vi "Counter output test.vi"() -> ()   [LabVIEW 2013]
uses:
  <vilib>/DAQmx/create/channels.llb/DAQmx Create Channel (CO-Pulse Generation-Time).vi
  <vilib>/DAQmx/configure/timing.llb/DAQmx Timing (Implicit).vi
  <resource>/objmgr/daqmx.rc
panel:
  out "CO.Count":u32
  in  "counter":tag caption="计数器"
  in  "low time":dbl=0.01 caption="低时间" format="%.6f"
  in  "high time":dbl=0.01 caption="高时间" format="%.6f"
  in  "CO.Pulse.Term":tag
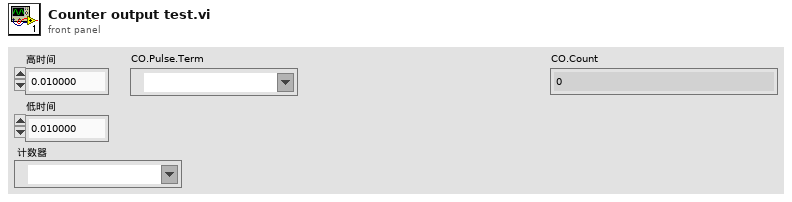
[diagram p1: front panel]
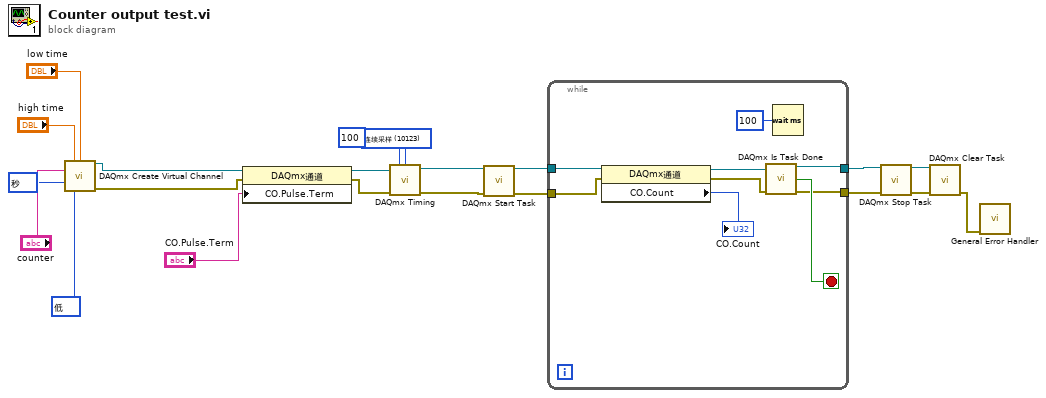
[diagram p0: block diagram]
diagram:
  w2 = 10214 items=["高"=10192, "低"=10214] ("idle state")
  w5 = 10364 items=["秒"=10364] ("units")
  w21 = 10123 items=["有限采样"=10178, "连续采样"=10123, "硬件定时单点"=12522] ("sample mode")
  n1 = call-poly <vilib>:"DAQmx Create Virtual Channel.vi"("high time"="high time", "low time"="low time", "counter"="counter", "units"=w5, "idle state"=w2) -> ("task out"=w9:refnum<k21>, "error out"=w8:errorcluster)  [unwired: 9 in]
  n2 = property class="DAQmx通道"(reference=w9, error in=w8, "CO.Pulse.Term"="CO.Pulse.Term") -> (reference out=w20:refnum<k21>, error out=w19:errorcluster)
  n3 = call-poly <vilib>:"DAQmx Timing.vi"("task/channels in"=w20, "sample mode"=w21, "samples per channel"=100, "error in"=w19) -> ("task out"=w18:refnum<k21>, "error out"=w10:errorcluster)  [unwired: 10 in]
  n4 = call <vilib>:"DAQmx Start Task.vi"("task/channels in"=w18, "error in"=w10) -> ("task out"=w17:refnum<k21>, "error out"=w16:errorcluster)  [unwired: 12 in]
  n5 = while {
    tunnel: w17 -> [w26]
    tunnel: w16 -> [w23]
    tunnel: [w30] -> w13
    tunnel: [w27] -> w12
    stop <- w29 stop-if-true
    n6 = property class="DAQmx通道"(reference=w26, error in=w23) -> (reference out=w25:refnum<k21>, error out=w24:errorcluster, "CO.Count"=→"CO.Count":u32)
    n7 = call <vilib>:"DAQmx Is Task Done.vi"("task/channels in"=w25, "error in"=w24) -> ("task out"=w30:refnum<k21>, "task done?"=w29:bool, "error out"=w27:errorcluster)  [unwired: 11 in]
    n8 = Wait (ms)(milliseconds to wait=u32 100 ("等待时间（毫秒）")) -> ()  [unwired: 1 out]
  }
  n9 = call <vilib>:"DAQmx Stop Task.vi"("task/channels in"=w13, "error in"=w12) -> ("task out"=w15:refnum<k21>, "error out"=w14:errorcluster)  [unwired: 12 in]
  n10 = call <vilib>:"DAQmx Clear Task.vi"("task in"=w15, "error in"=w14) -> ("error out"=w11:errorcluster)  [unwired: 13 in]
  n11 = call <vilib>:"General Error Handler.vi"("error in (no error)"=w11) -> ()  [unwired: 10 in, 5 out]
